vi "TSPopup.Initialize.vi"(8 "error in (no error)":errorcluster, 9 "Font Size":u32, 11 "Popup Cluster Ref":refnum<vi>) -> (0 "error out":errorcluster, 3 "Popup Event":refnum<user-event>)   [LabVIEW 2013]
doc: "Initializes the Type Sensitive Popup. Needs to be run at the beginning of the program.\n\n<B>Popup Cluster Ref</B> - Reference to the Popup Cluster which needs to be placed on the Front Panel of the VI. (cluster can be placed anywhere, but must be frontmost)\n<B>Font Size</B> - Sets the font size of popups with text.\n\n<B>Popup Event</B> - User Event reference. This must be registered by an Event Structure. It will fire when the popup data entry is complete.\n\nType Sensitive Popup \nCopyright © 2007, J. David Saunders\nAll rights reserved."
uses:
  Private/TSPopup.Popup Results.ctl
  Private/TSPopup.Popup Operation.ctl
panel:
  # "Type Sensitive Popup \nCopyright © 2007, J. David Saunders\nAll rights reserved."
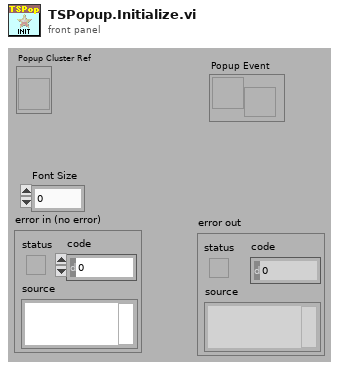
[diagram p1: front panel]
types:
  T1 = typedef "TSPopup.Popup Operation.ctl" = enum16{"Show", "Initialize", "Close", "Popup Done", "Register a Location's Type", "Retrieve Location's Type"}
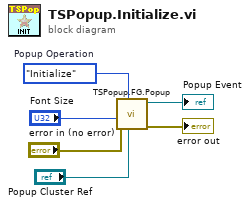
[diagram p0: block diagram]
diagram:
  w6 = TSPopup.Popup_Operation."Initialize"  # Popup Operation
  n1 = call "TSPopup.FG.Popup.vi"("Popup Cluster Ref"="Popup Cluster Ref", "Popup Operation"=w6, "error in (no error)"="error in (no error)", "Font Size"="Font Size") -> ("error out"=→"error out":errorcluster, "Popup Event"=→"Popup Event":refnum<user-event>)  [unwired: 4 in, 2 out]
